vi "broadcastTopic.vi"(8 "error in (no error)":errorcluster, 9 "Message":string, 10 "Topic":string, 11 "Module ID":i32=-1) -> (0 "error out":errorcluster)   [LabVIEW 2017, in "MQTT.lvlib"]
doc: "broadcasts the message received by MQTT client\n_____\nCreated using Delacor QMH Event Scripter 4.2.1.88."
uses:
  MQTT.lvlib
  broadcastTopic Argument--cluster.ctl
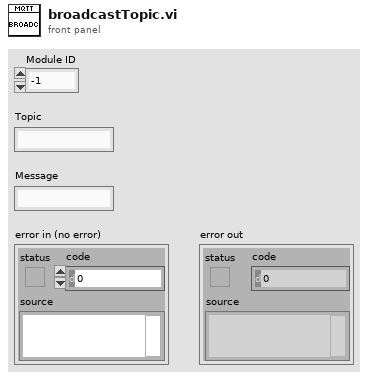
[diagram p1: front panel]
types:
  T1 = typedef "MQTT.lvlib/broadcastTopic Argument--cluster.ctl" = cluster{"Module ID":i32, "Topic":string, "Message":string}
  T2 = typedef "MQTT.lvlib/Request Events--cluster.ctl" = cluster{"Stop Module":refnum<user-event>, "Show Panel":refnum<user-event>, "Hide Panel":refnum<user-event>, "Show Diagram":refnum<user-event>, "Get Module Execution Status":refnum<user-event>, "Configure":refnum<user-event>, "Connect":refnum<user-event>, "disconnect":refnum<user-event>, "Subscrie":refnum<user-event>, "unsubscribe":refnum<user-event>, "Publish":refnum<user-event>, "Register Event":refnum<user-event>, "broadcastTopic":refnum<user-event>}
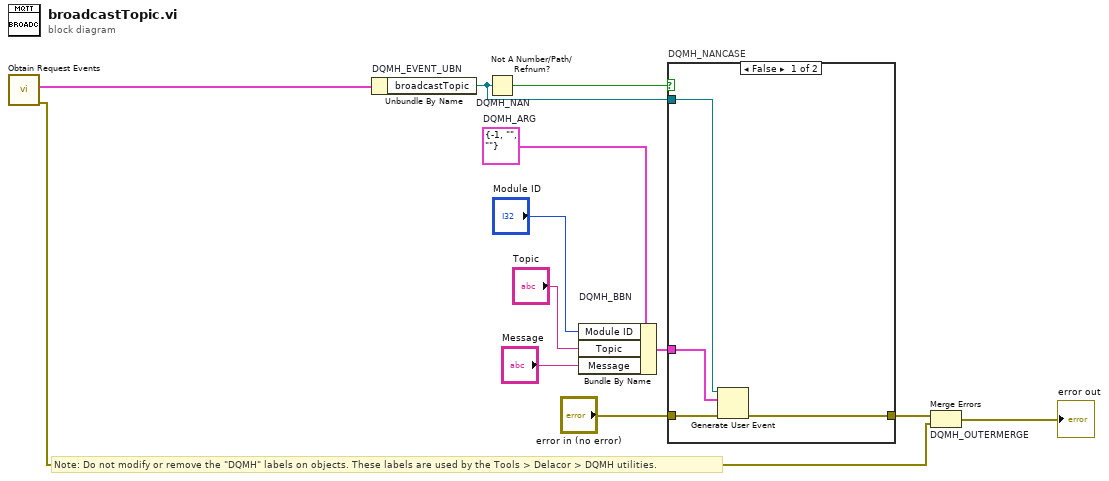
[diagram p0: block diagram]
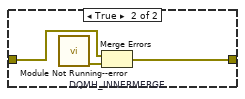
[diagram p2: hidden frame]
diagram:
  w6 = T1 {"Module ID"=-1, "Topic"="", "Message"=""}  # DQMH_ARG
  # "Note: Do not modify or remove the \"DQMH\" labels on objects. These labels are used by the Tools > Delacor > DQMH utilities."
  n1 = call "Obtain Request Events.vi"() -> ("error out"=w2:errorcluster, "MQTT Request Events"=w1:T2)  [unwired: 10 in]
  n2 = Unbundle By Name "DQMH_EVENT_UBN"(w1) -> ("broadcastTopic"=w8:refnum<user-event>)
  n3 = Not A Number/Path/Refnum? "DQMH_NAN"(number/path/refnum=w8) -> (NaN/Path/Refnum?=w9:bool)
  n4 = Bundle By Name "DQMH_BBN"(cluster=w6, "Module ID"="Module ID", "Topic"="Topic", "Message"="Message") -> (w10:T1)
  n5 = case "DQMH_NANCASE" shown="False" w9 {
    tunnel: "error in (no error)" -> [w16 w19]
    tunnel: [w15 w18] -> w7
    tunnel: w8 -> [w14 _]
    tunnel: w10 -> [w13 _]
    frame False {
      n6 = Generate User Event(user event=w14, event data cluster=w13, error in=w16) -> (error out=w15:errorcluster)  [unwired: 1 in, 1 out]
    }
    frame True {
      n7 = call "Module Not Running--error.vi"() -> ("error out"=w17:errorcluster)  [unwired: 11 in]
      n8 = Merge Errors "DQMH_INNERMERGE"(w19, w17) -> (w18:errorcluster)
    }
  }
  n9 = Merge Errors "DQMH_OUTERMERGE"(w7, w2) -> (→"error out":errorcluster)
